vi "GLOBAL_Scaler_Data.vi"(3 "Data in":u32[](array[numeric]), 5 "State":enum16{"Initialise", "Write", "Read"}(ring)) -> (0 "Acquisition Time":dbl, 1 "Data Out":u32[](array[numeric]))   [LabVIEW 2014]
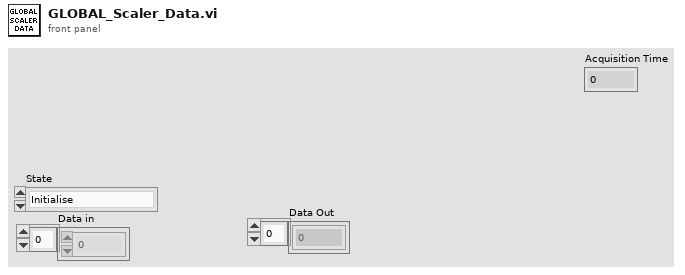
[diagram p1: front panel]
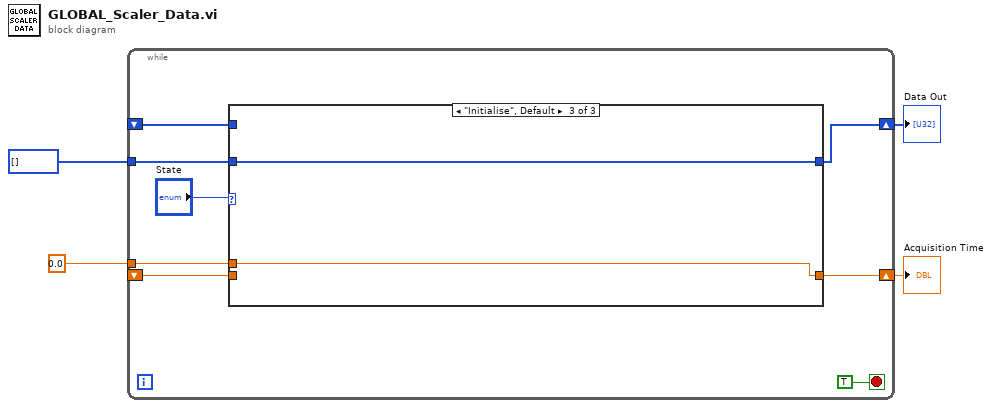
[diagram p0: block diagram]
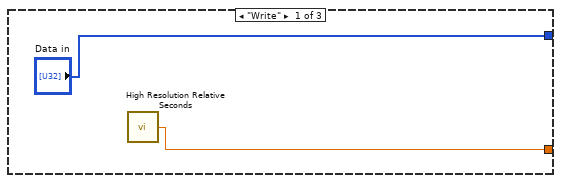
[diagram p2: hidden frame]
diagram:
  n1 = while {
    shift-right: [w9] -> w3
    shift-left: _ -> [w8]
    tunnel: u32[] [] ("Buff") -> [w10]
    shift-right: [w7] -> w2
    shift-left: _ -> [w6]
    tunnel: 0.0 ("relative seconds") -> [w5]
    stop <- TRUE stop-if-true
    n2 = case shown="\"Initialise\", Default" "State" {
      tunnel: w10 -> [_ _ w18]
      tunnel: ["Data in" w16 w18] -> w9
      tunnel: w8 -> [_ w16 _]
      tunnel: [w13 w15 w17] -> w7
      tunnel: w6 -> [_ w15 _]
      tunnel: w5 -> [_ _ w17]
      frame "Write" {
        n3 = call <vilib>:"High Resolution Relative Seconds.vi"() -> ("relative seconds"=w13:dbl)
      }
      frame "Read" {
      }
      frame "Initialise", Default {
      }
    }
  }
  "Data Out" <- w3
  "Acquisition Time" <- w2
